vi "basic tank drive.vi"   [LabVIEW 2010, in "Tank Robot.lvrbt"]
uses:
  Tank Robot.lvrbt
  <vilib>/NXT/NXTIO Xnodes/AddressXNode/NXTIOAddress.xnode
  <vilib>/NXT/Subs/MotorXNode.DC Motor Type.ctl
  <vilib>/NXT/Subs/MotorXNode.1DCMotor.ctl
  <vilib>/NXT/Subs/LVHSConnector.ctl
  <vilib>/NXT/NXTIO Xnodes/NXTIOXNode/NXTIO.xnode
  <vilib>/FTC/FTC Calculate Drive Power - Tank.vi
  <vilib>/NXT/NXTIO Xnodes/NXTIONodeSubVIs/TETRIX IO Move DC Motors.vi
types:
  T1 = typedef "FTC ControllerState.ctl" = cluster{"Left X":i8, "Left Y":i8, "Right X":i8, "Right Y":i8, "Button Encoding 9-12":u8, "Button Encoding 1-8":u8, "POV":T2}
  T2 = typedef "FTC POVState.ctl" = i8
  T3 = typedef "MotorXNode.DC Motor Type.ctl" = enum16{"DC Motor"}
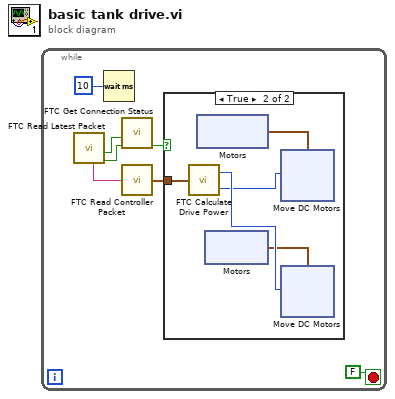
[diagram p0: block diagram]
diagram:
  n1 = while {
    stop <- FALSE stop-if-true
    n2 = call <vilib>:"FTC Read Latest Packet.vi"() -> ("Packet Received?"=w4:bool, "Stopped?"=w5:bool, "Controller 1"=w2:string)  [unwired: 6 in, 3 out]
    n3 = Wait (ms)(milliseconds to wait=u32 10) -> ()  [unwired: 1 out]
    n4 = call <vilib>:"FTC Get Connection Status.vi"("Packet Received?"=w4, "Stopped?"=w5) -> ("Online?"=w3:bool)  [unwired: 6 in, 2 out]
    n5 = call <vilib>:"FTC Read Controller Packet.vi"("Packet"=w2) -> ("Controller State"=w1:T1)  [unwired: 4 in]
    n6 = case shown="True" w3 {
      tunnel: w1 -> [_ w12]
      frame False {
      }
      frame True {
        n7 = call-poly <vilib>:"FTC Calculate Drive Power.vi"("Controller State"=w12) -> ("Right Motor Power"=w10:i8, "Left Motor Power"=w11:i8)  [unwired: 3 in]
        n8 = xnode "Motors"() -> ("DC Motor"=w8:cluster{"DC Motor":T3, "Address":i16})
        n9 = xnode "Motors"() -> ("DC Motor"=w9:cluster{"DC Motor":T3, "Address":i16})
        n10 = xnode "Move DC Motors"("Power/Speed 1"=w10, "Motors"=w8) -> ()  [unwired: 1 in, 1 out]
        n11 = xnode "Move DC Motors"("Power/Speed 1"=w11, "Motors"=w9) -> ()  [unwired: 1 in, 1 out]
      }
    }
  }
